vi "Plot.vi"(0 "SigMan in":refnum<class "SignalManager.lvclass">, 1 "Graph":refnum<vi>, 2 "VI":refnum<vi>, 5 "Array":dbl[][](array[numeric]), 7 "By channel":bool, 9 "Normalize":bool=TRUE, 11 "error in (no error)":errorcluster, 12 "Names":string[](array[string])) -> (4 "SigMan out":refnum<class "SignalManager.lvclass">, 15 "error out":errorcluster)   [LabVIEW 2020, in "SignalManager.lvclass"]
uses:
  SignalManager.lvclass
  SignalManager.lvclass/SignalManager.ctl
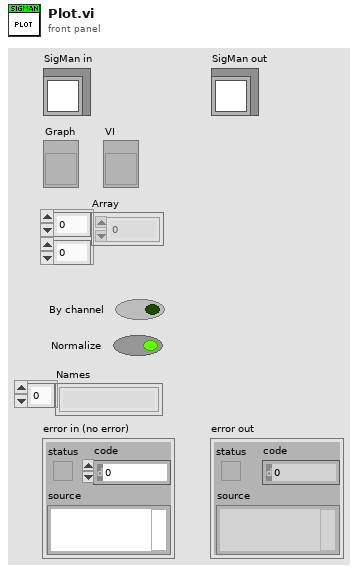
[diagram p1: front panel]
types:
  T1 = enum16{"User", "Prism", "Kelly", "Dark2", "Sequential", "Hue"}
  T2 = cluster{"Name":string, "Color":u32, "Style":u8, "Point Style":u8, "Name Visible":bool, "Allow Drag":bool, "Annotation Mode":u32, "Plot":i32, "Index":i32, "Position":cluster{"X":dbl, "Y":dbl}, "X Scale":u32, "Y Scale":u32, "Show Arrow":bool, "Lock Name":bool, "Plot Area":i32, "Label Offset":cluster{"X":dbl, "Y":dbl}}
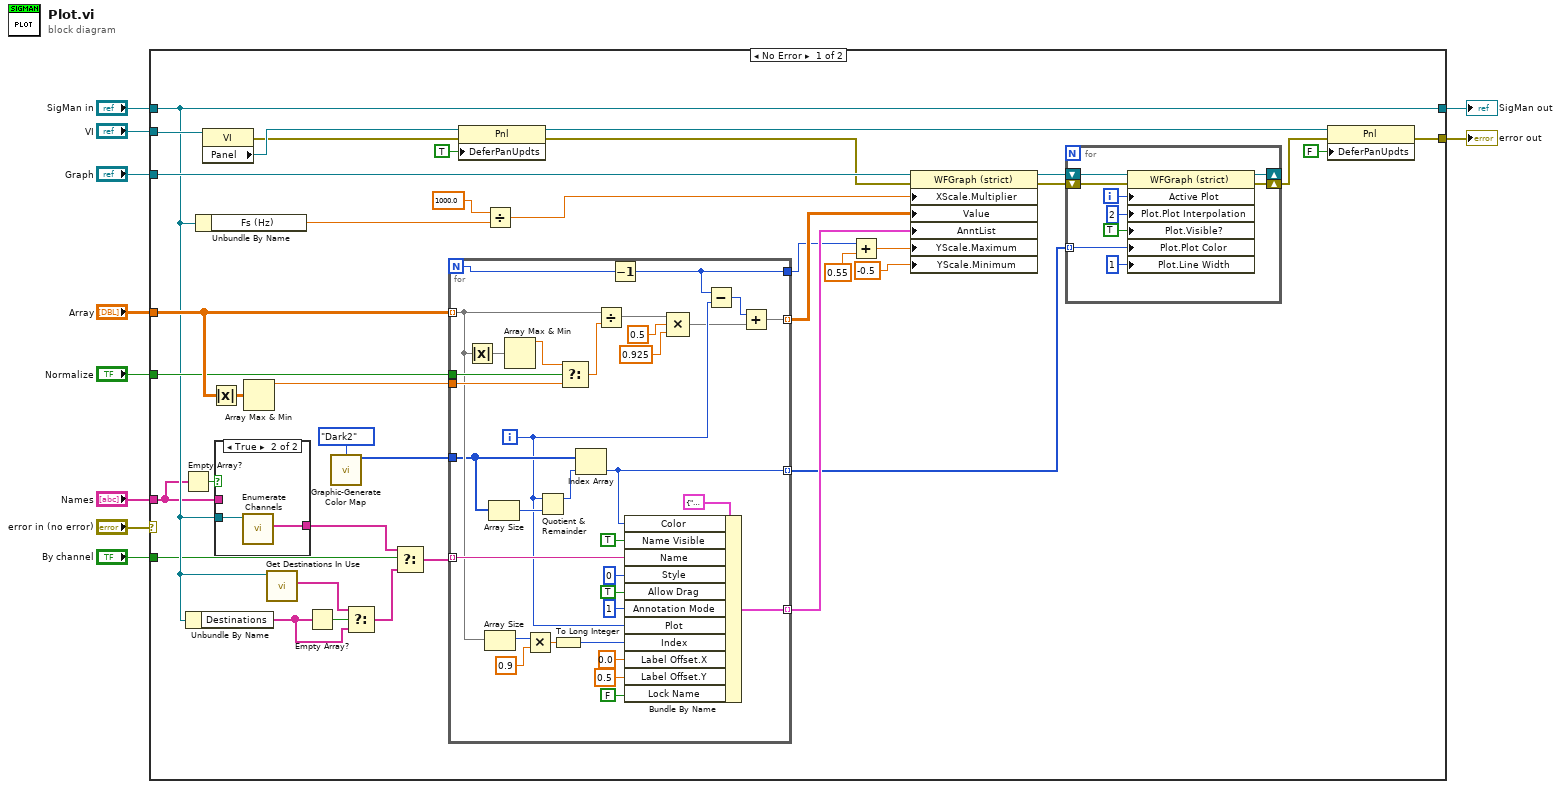
[diagram p0: block diagram]
diagram:
  n1 = case shown="No Error" "error in (no error)" {
    selector: "error in (no error)" -> [_ w95]
    tunnel: [w35 w95] -> w9
    tunnel: [w17 w94] -> w7
    tunnel: "SigMan in" -> [w17 w94]
    tunnel: "Array" -> [w47 _]
    tunnel: "Normalize" -> [w44 _]
    tunnel: "Graph" -> [w43 _]
    tunnel: "VI" -> [w27 _]
    tunnel: "By channel" -> [w16 _]
    tunnel: "Names" -> [w12 _]
    frame No Error {
      n2 = Empty Array?(array=w12) -> (empty?=w11:bool)
      n3 = Unbundle By Name(w17) -> ("Destinations"=w20:string[])
      n4 = Unbundle By Name(w17) -> ("Fs (Hz)"=w41:dbl)
      n5 = property class="VI"(reference=w27) -> (error out=w25:errorcluster, "Panel"=w26:refnum<vi>)  [unwired: 1 in, 1 out]
      n6 = Absolute Value(x=w47) -> (abs(x)=w46:dbl[][])
      n7 = case shown="True" w11 {
        tunnel: w17 -> [_ w51]
        tunnel: [w49 w50] -> w15
        tunnel: w12 -> [w49 _]
        frame False {
        }
        frame True {
          n8 = call "Enumerate Channels.vi"("SignalManager in"=w51) -> ("Names"=w50:string[])  [unwired: 8 in, 2 out]
        }
      }
      n9 = Array Max & Min(array=w46) -> (max value=w45:dbl)  [unwired: 3 out]
      n10 = call "Get Destinations In Use.vi"("SigMan in"=w17) -> ("Destinations in use"=w22:string[])  [unwired: 8 in, 2 out]
      n11 = Empty Array?(array=w20) -> (empty?=w21:bool)
      n12 = call "Graphic-Generate Color Map.vi"("Map"=T1."Dark2") -> ("Colors"=w28:u32[])  [unwired: 14 in]
      n13 = Select(t=w22, s=w21, f=w20) -> (s? t:f=w13:string[])
      n14 = Select(t=w15, s=w16, f=w13) -> (s? t:f=w14:string[])
      n15 = for {
        N -> [w70]
        tunnel: w47 -> [w77] mode=indexing
        tunnel: w45 -> [w90]
        tunnel: w44 -> [w92]
        tunnel: [w87] -> w42 mode=indexing
        tunnel: w14 -> [w78] mode=indexing
        tunnel: [w80] -> w34 mode=indexing
        tunnel: [w71] -> w30 mode=indexing
        tunnel: w28 -> [w72]
        tunnel: [w66] -> w24
        i -> [w69]
        n16 = Absolute Value(x=w77) -> (abs(x)=w93:dbl[])
        n17 = Array Size(array=w77) -> (size(s)=w65:i32)
        n18 = Array Size(array=w72) -> (size(s)=w74:i32)
        n19 = Array Max & Min(array=w93) -> (max value=w91:dbl)  [unwired: 3 out]
        n20 = Multiply(x=w65, y=0.9) -> (x*y=w64:dbl)
        n21 = Quotient & Remainder(x=w69, y=w74) -> (x-y*floor(x/y)=w73:i32)  [unwired: 1 out]
        n22 = To Long Integer(number=w64) -> (32bit integer=w62:i32)
        n23 = Select(t=w91, s=w92, f=w90) -> (s? t:f=w89:dbl)
        n24 = Index Array(array=w72, index=w73) -> (element=w71:u32)
        n25 = Divide(x=w77, y=w89) -> (x/y=w88:dbl[])
        n26 = Decrement(x=w70) -> (x-1=w66:i32)
        n27 = Bundle By Name(cluster=T2 {"Name"="", "Color"=0, "Style"=0, "Point Style"=0, "Name Visible"=FALSE, "Allow Drag"=FALSE, "Annotation Mode"=0, "Plot"=0, "Index"=0, "Position"={"X"=0.0, "Y"=0.0}, "X Scale"=0, "Y Scale"=0, "Show Arrow"=FALSE, "Lock Name"=FALSE, "Plot Area"=0, "Label Offset"={"X"=0.0, "Y"=0.0}} ("new element/subarray"), "Color"=w71, "Name Visible"=TRUE, "Name"=w78, "Style"=u8 0, "Allow Drag"=TRUE, "Annotation Mode"=u32 1, "Plot"=w69, "Index"=w62, "Label Offset.X"=0.0, "Label Offset.Y"=0.5, "Lock Name"=FALSE) -> (w80:T2)
        n28 = Compound Arithmetic op=MULTIPLY(w88, 0.5, 0.925) -> (w68:dbl[])
        n29 = Subtract(x=w66, y=w69) -> (x-y=w67:i32)
        n30 = Add(x=w67, y=w68) -> (x+y=w87:dbl[])
      }
      n31 = property class="Pnl"(reference=w26, error in=w25, "DeferPanUpdts"=TRUE ("Defer Panel Updates")) -> (reference out=w36:refnum<vi>, error out=w38:errorcluster)
      n32 = Divide(x=1000.0, y=w41) -> (x/y=w39:dbl)
      n33 = Add(x=w24, y=0.55 ("Y Scale.Range:Minimum")) -> (x+y=w19:dbl)
      n34 = property class="WFGraph (strict)"(reference=w43, error in=w38, "XScale.Multiplier"=w39, "Value"=w42, "AnntList"=w34, "YScale.Maximum"=w19, "YScale.Minimum"=-0.5 ("Y Scale.Range:Minimum")) -> (reference out=w33:refnum<vi>, error out=w32:errorcluster)
      n35 = for {
        shift-right: [w58] -> w31
        shift-left: w32 -> [w59]
        shift-right: [w56] -> _
        shift-left: w33 -> [w60]
        tunnel: w30 -> [w52] mode=indexing
        i -> [w55]
        n36 = property class="WFGraph (strict)"(reference=w60, error in=w59, "Active Plot"=w55, "Plot.Plot Interpolation"=u8 2, "Plot.Visible?"=TRUE ("Plot.Visible"), "Plot.Plot Color"=w52, "Plot.Line Width"=u8 1) -> (reference out=w56:refnum<vi>, error out=w58:errorcluster)
      }
      n37 = property class="Pnl"(reference=w36, error in=w31, "DeferPanUpdts"=FALSE ("Defer Panel Updates")) -> (error out=w35:errorcluster)  [unwired: 1 out]
    }
    frame Error {
    }
  }
  "error out" <- w9
  "SigMan out" <- w7
